vi "H-Drive Motors+Pneumatics.vi"(7 "Manual Mode":bool, 8 "Buttons[0]":bool, 9 "Buttons[3]":bool, 10 "Axes[3]":dbl, 11 "Axes[2]":dbl) -> (3 "H Drive Up":bool)   [LabVIEW 2015]
uses:
  <vilib>/Rock Robotics/WPI/Solenoid/Deprecated/WPI_SolenoidSetBool.vi
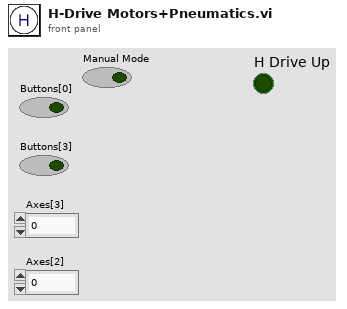
[diagram p1: front panel]
types:
  T1 = typedef "WPI_MotorControlDeviceRef.ctl" = cluster{"DeviceStatus":errorcluster, "Type":T2, "PWM":cluster{"PWM Channel":T3, "DeadBand":T4}, "CAN":cluster{"Device Number":u8, "Control Mode":T5, "Semaphore":T6, "Max Vout":dbl, "TalonSRX Control Mode":T7}, "Invert":bool}
  T2 = typedef "WPI_MotorControlType.ctl" = enum16{"PWM", "CAN", "CANTalonSRX"}
  T3 = typedef "FPGA_DIOPWMChannel.ctl" = enum8{"PWM 0", "PWM 1", "PWM 2", "PWM 3", "PWM 4", "PWM 5", "PWM 6", "PWM 7", "PWM 8", "PWM 9", "PWM MXP 0", "PWM MXP 1", "PWM MXP 2", "PWM MXP 3", "PWM MXP 4", "PWM MXP 5", "PWM MXP 6", "PWM MXP 7", "PWM MXP 8", "PWM MXP 9", "Invalid"}
  T4 = typedef "WPI_PWMDeadband.ctl" = cluster{"Name":string, "maxPositivePwm":i32, "minPositivePwm":i32, "centerPwm":i32, "maxNegativePwm":i32, "minNegativePwm":i32, "angularRange":u16}
  T5 = typedef "WPI_CANJaguar_ControlMode.ctl" = enum8{"Percent VBus", "Current", "Speed", "Position", "Voltage"}
  T6 = typedef "Semaphore RefNum" = refnum<k1>
  T7 = typedef "WPI_CANTalonSRX_APIControlMode.ctl" = enum8{"Percent VBus", "Speed", "Position", "Slave", "Unchanged / Invalid", "Voltage Compensation", "Current", "Motion Profile"}
  T8 = typedef "WPI_SolenoidDevRef.ctl" = cluster{"DevStatus":errorcluster, "Pneumatics Control Module":u8, "Forward Solenoid Channel":T9, "Reverse Solenoid Channel":T9}
  T9 = typedef "WPI_SolenoidChannel.ctl" = enum8{"Solenoid 0", "Solenoid 1", "Solenoid 2", "Solenoid 3", "Solenoid 4", "Solenoid 5", "Solenoid 6", "Solenoid 7", "Invalid"}
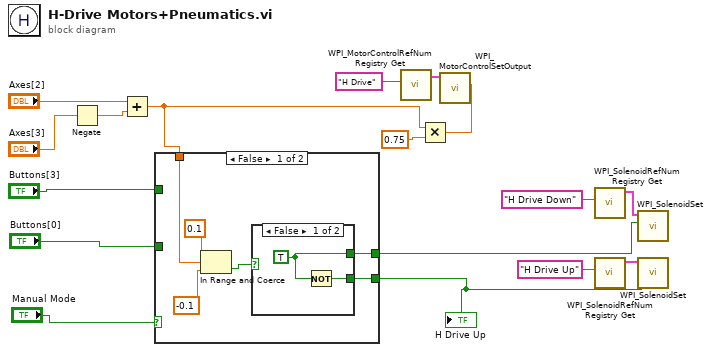
[diagram p0: block diagram]
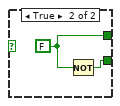
[diagram p2: hidden frame]
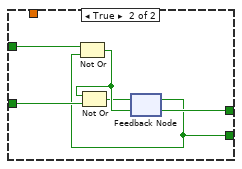
[diagram p3: hidden frame]
diagram:
  n1 = Negate(x="Axes[3]") -> (-x=w5:dbl)
  n2 = Add(x="Axes[2]", y=w5) -> (x+y=w2:dbl)
  n3 = case shown="False" "Manual Mode" {
    tunnel: "Buttons[0]" -> [_ w32]
    tunnel: "Buttons[3]" -> [_ w31]
    tunnel: [w22 w30] -> w11
    tunnel: [w23 w29] -> w10
    tunnel: w2 -> [w18 _]
    frame False {
      n4 = In Range and Coerce(upper limit=0.1, x=w18, lower limit=-0.1) -> (In Range?=w21:bool)  [unwired: 1 out]
      n5 = case shown="False" w21 {
        tunnel: [w25 w27] -> w23
        tunnel: [w24 w26] -> w22
        frame False {
          w24 = TRUE
          n6 = Not(x=w24) -> (.not. x?=w25:bool)
        }
        frame True {
          w26 = FALSE
          n7 = Not(x=w26) -> (.not. x?=w27:bool)
        }
      }
    }
    frame True {
      n8 = feedback #1() -> (w29:bool)  [unwired: 1 in]
      n9 = Not Or(1:w29, 2:w31) -> (0:w30:bool)
      n10 = Not Or(1:w32, 2:w30) -> (0:w28:bool)
      n11 = feedback-in #1(w28) -> ()
    }
  }
  "H Drive Up" <- w10
  n12 = call <vilib>:"WPI_MotorControlRefNum Registry Get.vi"("refnum name"="H Drive") -> ("MotorControlDevRef"=w4:T1)  [unwired: 9 in, 1 out]
  n13 = Multiply(x=w2, y=0.75) -> (x*y=w9:dbl)
  n14 = call <vilib>:"WPI_MotorControlSetOutput.vi"("Output"=w9, "MotorControlDevRef"=w4) -> ()  [unwired: 7 in, 3 out]
  n15 = call <vilib>:"WPI_SolenoidRefNum Registry Get.vi"("refnum name"="H Drive Down") -> ("SolenoidDevRef"=w13:T8)  [unwired: 9 in, 1 out]
  n16 = call <vilib>:"WPI_SolenoidRefNum Registry Get.vi"("refnum name"="H Drive Up") -> ("SolenoidDevRef"=w14:T8)  [unwired: 9 in, 1 out]
  n17 = call-poly <vilib>:"WPI_SolenoidSet.vi"("Value"=w11, "SolenoidDevRef"=w13) -> ()  [unwired: 8 in, 2 out]
  n18 = call-poly <vilib>:"WPI_SolenoidSet.vi"("Value"=w10, "SolenoidDevRef"=w14) -> ()  [unwired: 8 in, 2 out]
